vi "Packet_encode_FLT64.vi"(9 "FLT64_Value":dbl, 11 "RawData In":u8[](array[numeric])) -> (3 "RawData Out":u8[](array[numeric]))   [LabVIEW 2019, in "PhotonVisionLib.lvlib"]
doc: "Encode (or append) a double floating point value (FLT 64) at the end of an array of bytes. No conversion is actually done, the memory is just copied to the end of the array.\n\nInputs\n - RawData In -- Array of bytes to be appended to..\n - FLT64_Value -- Double floating point value.\n\nOutputs\n - RawData Out -- Array of bytes containing the appended value."
uses:
  PhotonVisionLib.lvlib
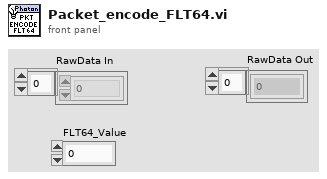
[diagram p1: front panel]
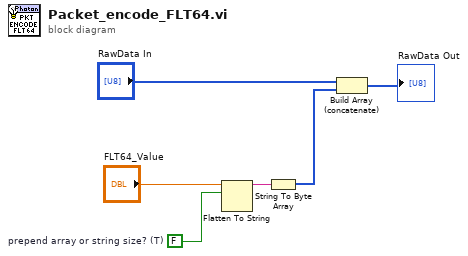
[diagram p0: block diagram]
diagram:
  w5 = FALSE  # prepend array or string size? (T)
  n1 = Flatten To String(anything="FLT64_Value", prepend array or string size? (T)=w5) -> (data string=w3:string)  [unwired: 2 in, 2 out]
  n2 = String To Byte Array(string=w3) -> (unsigned byte array=w2:u8[])
  n3 = Build Array (concatenate)("RawData In", w2) -> (→"RawData Out":u8[])
